vi "DEMO.vi"() -> ()   [LabVIEW 2012]
uses:
  Custom Def/Employee Info.ctl
  Custom Def/Salary Info.ctl
  Custom Def/Select Table.ctl
  Employee Class/Employee.lvclass
  System.Windows.Forms
panel:
  in  "Select Table":T1=enum."Salary"
  in  "Employees Salary Info":T2[](array[typedef])=[{"ID"=1305, "Working Days"=30.0, "Total Salary"=7200.0}, {"ID"=1201, "Working Days"=30.0, "Total Salary"=4050.0}]
  in  "停止":bool
  in  "DataGridView":refnum<k24>(container)
  in  "Employees Info":T3[](array[typedef])=[{"ID"=1201, "Name"="张燕", "Married"=FALSE, "Age"=20, "Sex"="Female", "Job"="秘书", "BirthDay"=timestamp(2815111959.1696 s since 1904-01-01)}, {"ID"=1305, "Name"="王磊", "Married"=TRUE, "Age"=35, "Sex"="Male", "Job"="技术部长", "BirthDay"=timestamp(2688717336.1618 s since 1904-01-01)}]
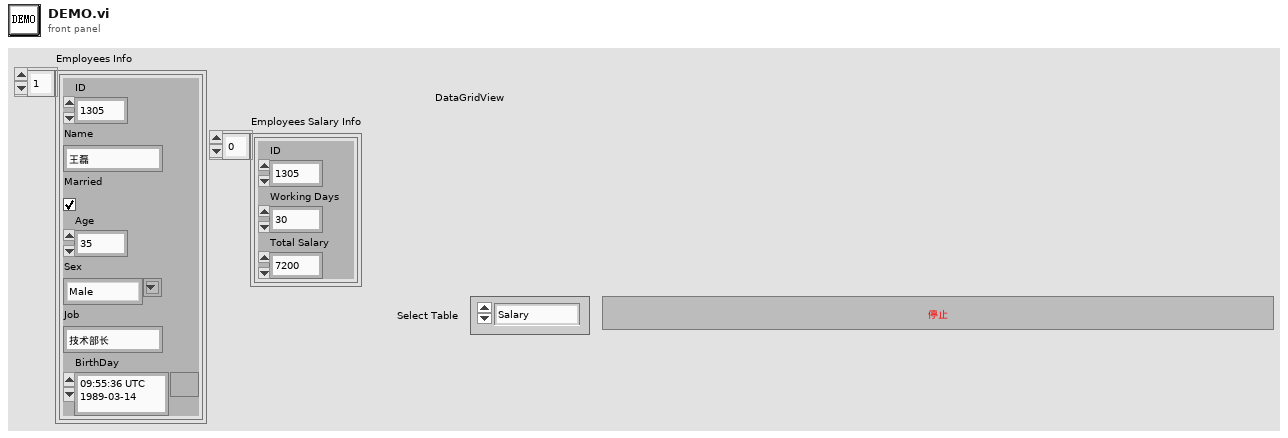
[diagram p1: front panel]
types:
  T1 = typedef "Select Table.ctl" = enum16{"Info", "Salary"}
  T2 = typedef "Salary Info.ctl" = cluster{"ID":u16, "Working Days":dbl, "Total Salary":dbl}
  T3 = typedef "Employee Info.ctl" = cluster{"ID":u16, "Name":string, "Married":bool, "Age":u8, "Sex":string, "Job":string, "BirthDay":timestamp}
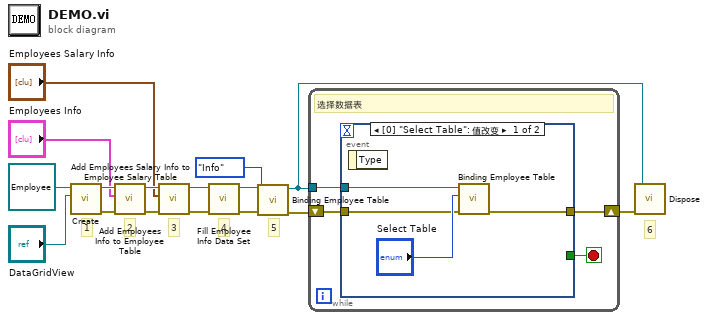
[diagram p0: block diagram]
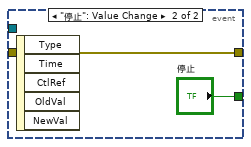
[diagram p2: hidden frame]
diagram:
  # "6"
  # "5"
  # "4"
  # "3"
  # "2"
  # "1"
  n1 = call "Create.vi"("DataGridView"="DataGridView", "Employee 输入"=refnum<class "Employee.lvclass"> refnum ("Employee.lvclass")) -> ("error out"=w15:errorcluster, "Employee 输出"=w14:refnum<class "Employee.lvclass">)  [unwired: 8 in]
  n2 = call "Add Employees Info to Employee Table.vi"("error in (no error)"=w15, "Employees Info"="Employees Info", "Employee 输入"=w14) -> ("error out"=w11:errorcluster, "Employee 输出"=w8:refnum<class "Employee.lvclass">)  [unwired: 7 in]
  n3 = call "Add Employees Salary Info to Employee Salary Table.vi"("error in (no error)"=w11, "Employees Salary Info"="Employees Salary Info", "Employee 输入"=w8) -> ("error out"=w10:errorcluster, "Employee 输出"=w9:refnum<class "Employee.lvclass">)  [unwired: 7 in]
  n4 = call "Fill Employee Info Data Set.vi"("error in (no error)"=w10, "Employee 输入"=w9) -> ("error out"=w4:errorcluster, "Employee 输出"=w5:refnum<class "Employee.lvclass">)  [unwired: 8 in]
  n5 = call "Binding Employee Table.vi"("error in (no error)"=w4, "Select Table"=Select_Table."Info", "Employee 输入"=w5) -> ("error out"=w3:errorcluster, "Employee 输出"=w1:refnum<class "Employee.lvclass">)  [unwired: 7 in]
  n6 = while {
    tunnel: w1 -> [w19]
    shift-right: [w18] -> w6
    shift-left: w3 -> [w17]
    stop <- w20 stop-if-true
    # "选择数据表"
    n7 = event shown="[0] \"Select Table\": 值改变" {
      selector: _ -> [_ _]
      dyn-events: _ -> [_ _]
      timeout: _ -> [_ _]
      tunnel: [_ "停止"] -> w20
      tunnel: w19 -> [w24 _]
      tunnel: w17 -> [w22 w25]
      tunnel: [w21 w25] -> w18
      event Value Change {
        n8 = event-data() -> ()  [unwired: 1 in, 1 out]
        n9 = call "Binding Employee Table.vi"("error in (no error)"=w22, "Select Table"="Select Table", "Employee 输入"=w24) -> ("error out"=w21:errorcluster)  [unwired: 7 in, 1 out]
      }
      event "停止": Value Change {
        n10 = event-data() -> ()  [unwired: 1 in, 5 out]
      }
    }
  }
  n11 = call "Dispose.vi"("error in (no error)"=w6, "Employee 输入"=w1) -> ()  [unwired: 8 in, 2 out]
